vi "RT to FPGA - Pan and Volume.vi"(7 "Track Controls":T1 {"Track 3"."Volume Settings"."Volume" scale=1.0..10.0; "Track 3"."Volume Settings"."Pan" scale=0.0..1.0; "Track 3"."Effects Settings"."Delay 2" scale=0.0..10.0; "Track 3"."Effects Settings"."Delay" scale=0.0..1.0; "Track 2"."Volume Settings"."Volume" scale=1.0..10.0; "Track 2"."Volume Settings"."Pan" scale=0.0..1.0; "Track 2"."Effects Settings"."Delay 2" scale=0.0..10.0; "Track 2"."Effects Settings"."Delay" scale=0.0..1.0; "Track 1"."Volume Settings"."Volume" scale=1.0..10.0; "Track 1"."Volume Settings"."Pan" scale=0.0..1.0; "Track 1"."Effects Settings"."Delay 2" scale=0.0..10.0; "Track 1"."Effects Settings"."Delay" scale=0.0..1.0; "Track 0"."Volume Settings"."Volume" scale=1.0..10.0; "Track 0"."Volume Settings"."Pan" scale=0.0..1.0; "Track 0"."Effects Settings"."Delay 2" scale=0.0..10.0; "Track 0"."Effects Settings"."Delay" scale=0.0..1.0}, 8 "error in":errorcluster, 11 "Refnum in":refnum<k20>) -> (0 "error out":errorcluster, 3 "Refnum out":refnum<k20>)   [LabVIEW 2014]
uses:
  Track Controls.ctl
  Track Settings.ctl
  Track Effects Settings.ctl
  Track Volume Settings.ctl
  <vilib>/Utility/error.llb/Error Cluster From Error Code.vi
  <vilib>/rvi/errors/niLvFpgaAdjustHostInterfaceError.vi
  <vilib>/rvi/interface/nirviReadWriteControl/nirviReadWriteControl.xnode
  NiFpgaLv.dll
  <vilib>/rvi/interface/Simulation/niFpgaSimulationCallBeginRW.vi
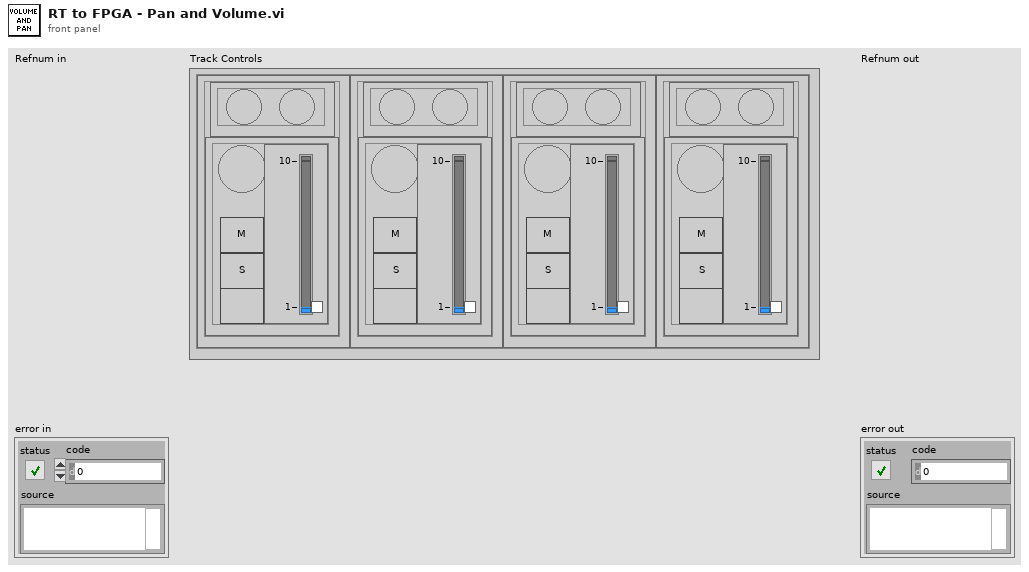
[diagram p1: front panel]
types:
  T1 = typedef "Track Controls.ctl" = cluster{"Track 0":T2, "Track 1":T2, "Track 2":T2, "Track 3":T2}
  T2 = typedef "Track Settings.ctl" = cluster{"Effects Settings":T3, "Volume Settings":T4}
  T3 = typedef "Track Effects Settings.ctl" = cluster{"Delay":dbl, "Delay 2":dbl}
  T4 = typedef "Track Volume Settings.ctl" = cluster{"Mute":bool, "Solo":bool, "Record":bool, "Pan":dbl, "Volume":dbl}
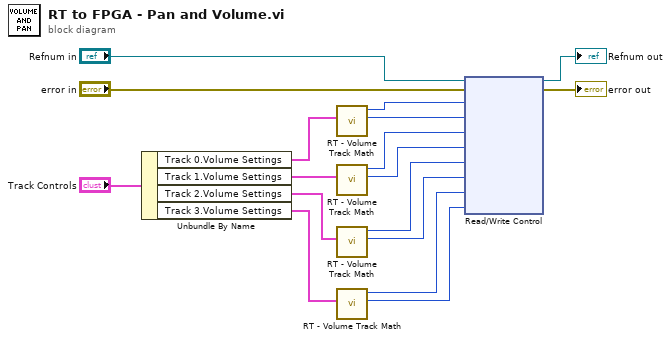
[diagram p0: block diagram]
diagram:
  n1 = Unbundle By Name("Track Controls") -> ("Track 0.Volume Settings"=w9:T4, "Track 1.Volume Settings"=w10:T4, "Track 2.Volume Settings"=w8:T4, "Track 3.Volume Settings"=w7:T4)
  n2 = call "RT - Volume Track Math.vi"("input cluster"=w9) -> ("Numeric"=w14:u16, "Numeric 2"=w15:u16)  [unwired: 9 in]
  n3 = call "RT - Volume Track Math.vi"("input cluster"=w10) -> ("Numeric"=w5:u16, "Numeric 2"=w6:u16)  [unwired: 9 in]
  n4 = call "RT - Volume Track Math.vi"("input cluster"=w8) -> ("Numeric"=w3:u16, "Numeric 2"=w4:u16)  [unwired: 9 in]
  n5 = call "RT - Volume Track Math.vi"("input cluster"=w7) -> ("Numeric"=w1:u16, "Numeric 2"=w2:u16)  [unwired: 9 in]
  n6 = xnode "Read/Write Control"("FPGA VI Reference In"="Refnum in", "error in"="error in", "Pan Left 0"=w15, "Pan Right 0"=w14, "Pan Left 1"=w6, "Pan Right 1"=w5, "Pan Left 2"=w4, "Pan Right 2"=w3, "Pan Left 3"=w2, "Pan Right 3"=w1) -> ("FPGA VI Reference Out"=→"Refnum out":refnum<k20>, "error out"=→"error out":errorcluster)
